vi "Read Teller.vi"(11 "TEMPLATE Msg in":refnum<class "TEMPLATE Msg.lvclass">) -> (2 "Teller":refnum<class "Teller.lvclass">)   [LabVIEW 2025, in "_Template.lvlib" / "Templates.lvlib" / "TEMPLATE Msg.lvlib" / "TEMPLATE Msg.lvclass"]
uses:
  TEMPLATE Msg.lvclass
  jettl/jettl/Teller/Teller/Teller.lvclass
  TEMPLATE Msg.lvclass/TEMPLATE Msg.ctl
panel:
  # "This front panel should not be manipulated."
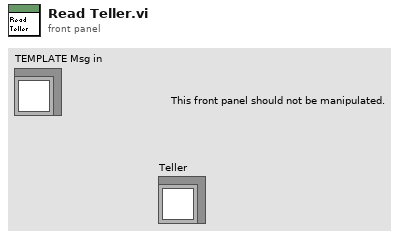
[diagram p1: front panel]
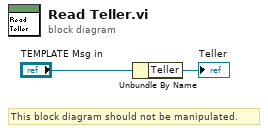
[diagram p0: block diagram]
diagram:
  # "This block diagram should not be manipulated."
  n1 = Unbundle By Name("TEMPLATE Msg in") -> ("Teller"=→"Teller":refnum<class "Teller.lvclass">)
